vi "displayResult.vi"(0 "HB_PollingAgent in":refnum<class "HB_PollingAgent.lvclass">, 11 "error in (no error)":errorcluster) -> (4 "HB_PollingAgent out":refnum<class "HB_PollingAgent.lvclass">, 15 "error out":errorcluster)   [LabVIEW 2009, in "HB_PollingAgent.lvlib" / "HB_PollingAgent.lvclass"]
uses:
  HB_PollingAgent.lvclass
  HB_PollingAgent.lvclass/HB_PollingAgent.ctl
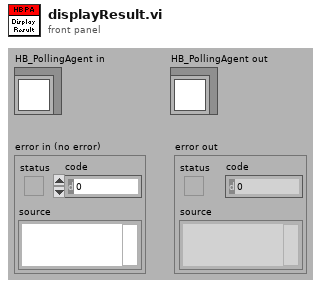
[diagram p1: front panel]
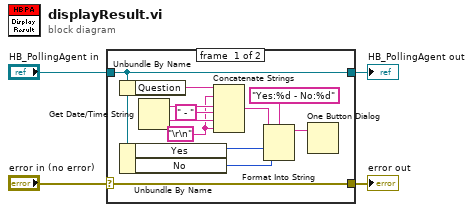
[diagram p0: block diagram]
diagram:
  n1 = case shown="No Error" "error in (no error)" {
    selector: "error in (no error)" -> [w16 w18]
    tunnel: [w16 w18] -> w3
    tunnel: [w6 w17] -> w1
    tunnel: "HB_PollingAgent in" -> [w6 w17]
    frame #0 {
      w7 = "\r\n"
      n2 = Unbundle By Name(w6) -> ("Question"=w5:string)
      n3 = Unbundle By Name(w6) -> ("Yes"=w11:u32, "No"=w10:u32)
      n4 = Get Date/Time String() -> (date string=w15:string, time string=w14:string)  [unwired: 3 in]
      n5 = Concatenate Strings(w5, w7, w15, " - " ("string"), w14, w7) -> (w12:string)
      n6 = Format Into String(format string="Yes:%d - No:%d", initial string=w12, w11, w10) -> (resulting string=w9:string)  [unwired: 1 in, 1 out]
      n7 = One Button Dialog(message=w9) -> ()  [unwired: 1 in, 1 out]
    }
    frame #1 {
    }
  }
  "error out" <- w3
  "HB_PollingAgent out" <- w1
